vi "expm.vi"(1 "ak":dbl, 2 "p":dbl) -> (0 "y":dbl)   [LabVIEW 2023]
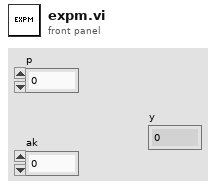
[diagram p1: front panel]
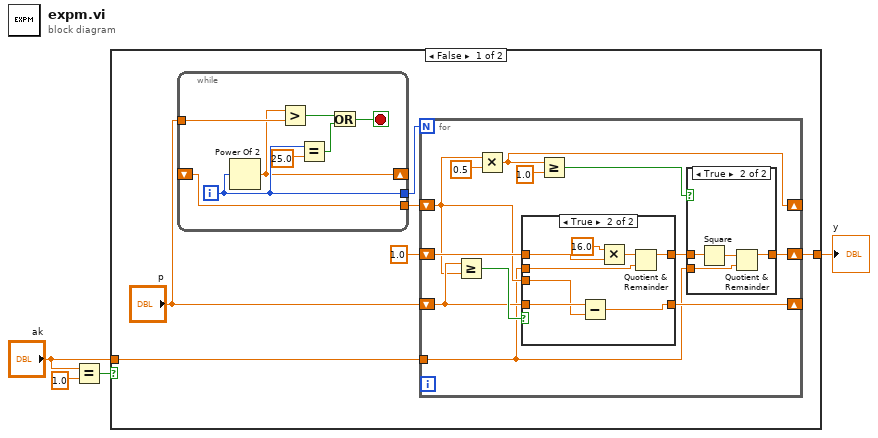
[diagram p0: block diagram]
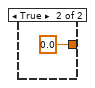
[diagram p4: hidden frame]
diagram:
  n1 = Equal?(x="ak", y=1.0) -> (x = y?=w1:bool)
  n2 = case shown="False" w1 {
    tunnel: [w7 0.0 ("y")] -> w4
    tunnel: "ak" -> [w6 _]
    frame False {
      n3 = while {
        tunnel: "p" -> [w45]
        tunnel: [w39] -> w9
        tunnel: [w40] -> w5
        shift-right: [w38] -> _
        shift-left: _ -> [w39]
        i -> [w40]
        stop <- w43 stop-if-true
        n4 = Power Of 2(x=w40) -> (2^x=w38:dbl)
        n5 = Greater?(x=w38, y=w45) -> (0:w42:bool)
        n6 = Equal?(x=w40, y=25.0) -> (x = y?=w41:bool)
        n7 = Or(x=w42, y=w41) -> (x .or. y?=w43:bool)
      }
      n8 = for {
        N: w5 -> [_]
        shift-right: [w20] -> _
        shift-left: "p" -> [w19]
        shift-right: [w16] -> _
        shift-left: w9 -> [w18]
        shift-right: [w12] -> w7
        shift-left: 1.0 ("y") -> [w21]
        tunnel: w6 -> [w11]
        n9 = Greater Or Equal?(x=w19, y=w18) -> (x >= y?=w22:bool)
        n10 = Multiply(x=w18, y=0.5) -> (x*y=w16:dbl)
        n11 = case shown="True" w22 {
          tunnel: w21 -> [w28 w36]
          tunnel: w18 -> [_ w32]
          tunnel: [w29 w34] -> w20
          tunnel: w19 -> [w29 w33]
          tunnel: [w28 w31] -> w13
          tunnel: w11 -> [_ w30]
          frame False {
          }
          frame True {
            n12 = Subtract(x=w33, y=w32) -> (x-y=w34:dbl)
            n13 = Multiply(x=16.0, y=w36) -> (x*y=w35:dbl)
            n14 = Quotient & Remainder(x=w35, y=w30) -> (x-y*floor(x/y)=w31:dbl)  [unwired: 1 out]
          }
        }
        n15 = Greater Or Equal?(x=w16, y=1.0) -> (x >= y?=w14:bool)
        n16 = case shown="True" w14 {
          tunnel: w13 -> [w23 w27]
          tunnel: [w23 w26] -> w12
          tunnel: w11 -> [_ w25]
          frame False {
          }
          frame True {
            n17 = Square(x=w27) -> (x^2=w24:dbl)
            n18 = Quotient & Remainder(x=w24, y=w25) -> (x-y*floor(x/y)=w26:dbl)  [unwired: 1 out]
          }
        }
      }
    }
    frame True {
    }
  }
  "y" <- w4
